vi "SECoP-simpleStringFromJSON.vi"(11 "String in":string) -> (3 "String 3":string)   [LabVIEW 2023, in "SECoP.lvlib"]
uses:
  SECoP.lvlib
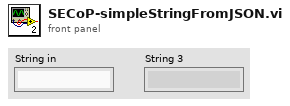
[diagram p1: front panel]
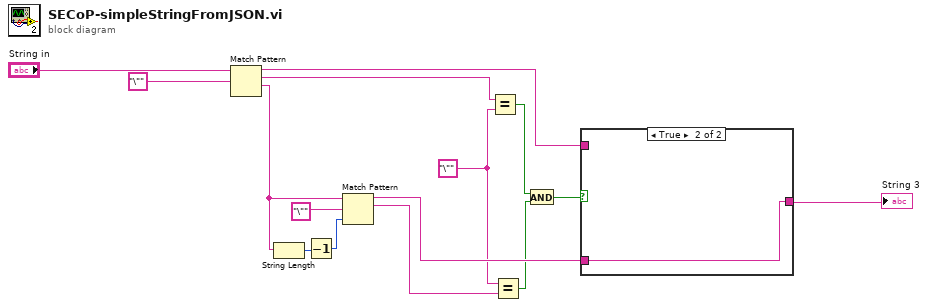
[diagram p0: block diagram]
diagram:
  w8 = "\""
  n1 = Match Pattern(string="String in", regular expression="\"") -> (before substring=w11:string, match substring=w9:string, after substring=w4:string)  [unwired: 1 in, 1 out]
  n2 = String Length(string=w4) -> (length=w3:i32)
  n3 = Decrement(x=w3) -> (x-1=w2:i32)
  n4 = Match Pattern(string=w4, regular expression="\"", offset (0)=w2) -> (before substring=w13:string, match substring=w10:string)  [unwired: 2 out]
  n5 = Equal?(x=w9, y=w8) -> (x = y?=w6:bool)
  n6 = Equal?(x=w8, y=w10) -> (x = y?=w5:bool)
  n7 = And(x=w6, y=w5) -> (x .and. y?=w7:bool)
  n8 = case shown="True" w7 {
    tunnel: w13 -> [_ w17]
    tunnel: w11 -> [w16 _]
    tunnel: [w16 w17] -> w12
    frame False {
    }
    frame True {
    }
  }
  "String 3" <- w12
